vi "VITester_Item_Interface.vi"() -> (3 "InterfaceTable":T1)   [LabVIEW 2009]
uses:
  API/Item_Interface.ctl
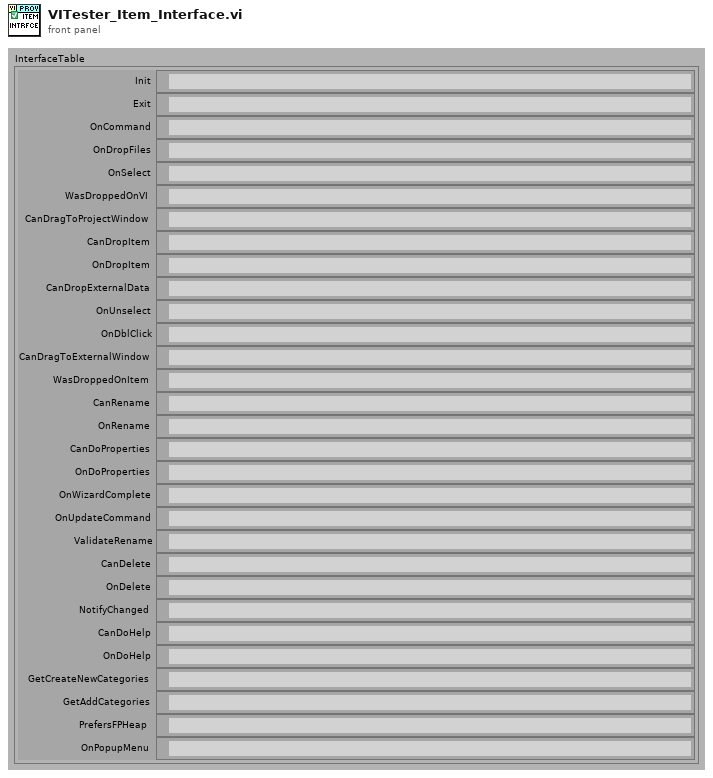
[diagram p1: front panel]
types:
  T1 = typedef "Item_Interface.ctl" = cluster{"Init":path, "Exit":path, "OnCommand":path, "OnDropFiles":path, "OnSelect":path, "WasDroppedOnVI":path, "CanDragToProjectWindow":path, "CanDropItem":path, "OnDropItem":path, "CanDropExternalData":path, "OnUnselect":path, "OnDblClick":path, "CanDragToExternalWindow":path, "WasDroppedOnItem":path, "CanRename":path, "OnRename":path, "CanDoProperties":path, "OnDoProperties":path, "OnWizardComplete":path, "OnUpdateCommand":path, "ValidateRename":path, "CanDelete":path, "OnDelete":path, "NotifyChanged":path, "CanDoHelp":path, "OnDoHelp":path, "GetCreateNewCategories":path, "GetAddCategories":path, "PrefersFPHeap":path, "OnPopupMenu":path}
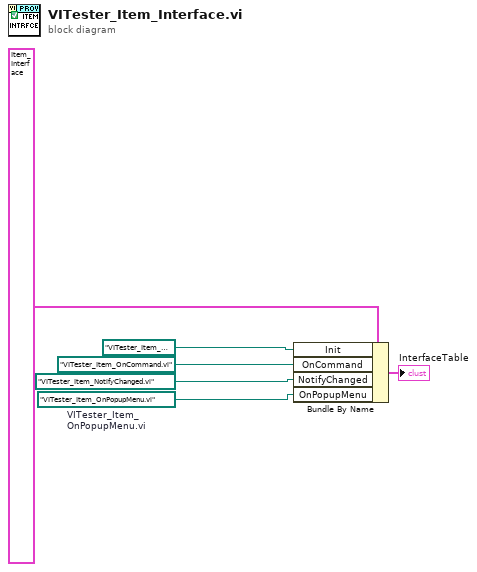
[diagram p0: block diagram]
diagram:
  w1 = path "VITester_Item_OnPopupMenu.vi"  # VITester_Item_OnPopupMenu.vi
  n1 = Bundle By Name(cluster=T1 {"Init"=path "", "Exit"=path "", "OnCommand"=path "", "OnDropFiles"=path "", "OnSelect"=path "", "WasDroppedOnVI"=path "", "CanDragToProjectWindow"=path "", "CanDropItem"=path "", "OnDropItem"=path "", "CanDropExternalData"=path "", "OnUnselect"=path "", "OnDblClick"=path "", "CanDragToExternalWindow"=path "", "WasDroppedOnItem"=path "", "CanRename"=path "", "OnRename"=path "", "CanDoProperties"=path "", "OnDoProperties"=path "", "OnWizardComplete"=path "", "OnUpdateCommand"=path "", "ValidateRename"=path "", "CanDelete"=path "", "OnDelete"=path "", "NotifyChanged"=path "", "CanDoHelp"=path "", "OnDoHelp"=path "", "GetCreateNewCategories"=path "", "GetAddCategories"=path "", "PrefersFPHeap"=path "", "OnPopupMenu"=path ""} ("InterfaceTable"), "Init"=path "VITester_Item_Init.vi", "OnCommand"=path "VITester_Item_OnCommand.vi", "NotifyChanged"=path "VITester_Item_NotifyChanged.vi", "OnPopupMenu"=w1) -> (→"InterfaceTable":T1)
